vi "BIN_PAQ_day_nums_2_filename.vi"(6 "num Stop":u64, 8 "error in":errorcluster, 9 "num Start":u64, 10 "ext":string, 11 "TableName":string) -> (0 "error out":errorcluster, 2 "FileNames":string[](array[string]))   [LabVIEW 2020, in "Sgraph_lib_V1.lvlib" / "DBAL-BIN.lvclass"]
doc: "Binary PAQ file: numeric file identifier to filename\n(array of 1 or two names)"
uses:
  DBAL-BIN.lvclass
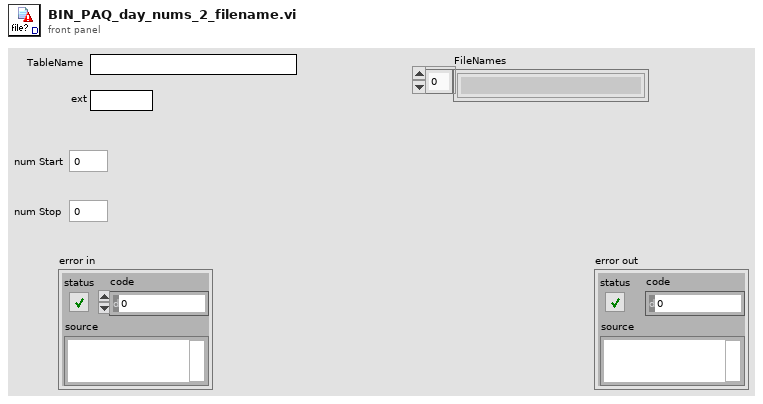
[diagram p1: front panel]
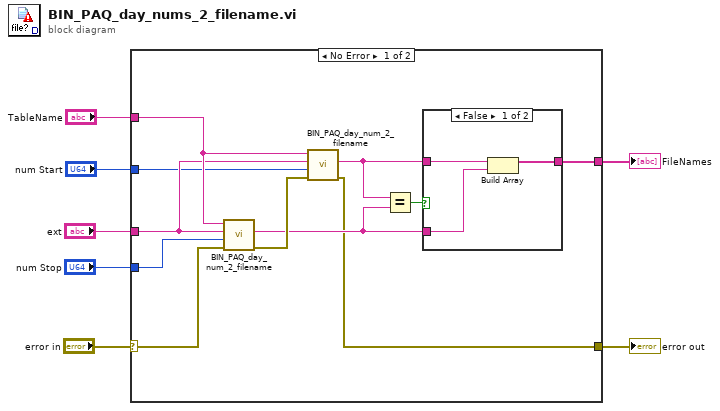
[diagram p0: block diagram]
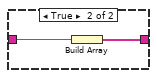
[diagram p2: hidden frame]
diagram:
  n1 = case shown="No Error" "error in" {
    selector: "error in" -> [w9 w24]
    tunnel: "TableName" -> [w18 _]
    tunnel: "ext" -> [w17 _]
    tunnel: "num Start" -> [w16 _]
    tunnel: "num Stop" -> [w15 _]
    tunnel: [w10 _] -> w3
    tunnel: [w8 w24] -> w1
    frame No Error {
      n2 = call "BIN_PAQ_day_num_2_filename.vi"("error in"=w9, "num"=w15, "ext"=w17, "TableName"=w18) -> ("error out"=w14:errorcluster, "FileName"=w11:string)  [unwired: 6 in]
      n3 = call "BIN_PAQ_day_num_2_filename.vi"("error in"=w14, "num"=w16, "ext"=w17, "TableName"=w18) -> ("error out"=w8:errorcluster, "FileName"=w12:string)  [unwired: 6 in]
      n4 = Equal?(x=w12, y=w11) -> (x = y?=w13:bool)
      n5 = case shown="False" w13 {
        tunnel: w12 -> [w21 w23]
        tunnel: [w20 w22] -> w10
        tunnel: w11 -> [w19 _]
        frame False {
          n6 = Build Array(w21, w19) -> (w20:string[])
        }
        frame True {
          n7 = Build Array(w23) -> (w22:string[])
        }
      }
    }
    frame Error {
    }
  }
  "FileNames" <- w3
  "error out" <- w1
